vi "Clear.vi"(8 "error in (no error)":errorcluster, 11 "Process In":refnum<class "Process.lvclass">) -> (0 "error out":errorcluster, 3 "Process Out":refnum<class "Process.lvclass">)   [LabVIEW 2020, in "Process.lvclass"]
doc: "Clears any resorces allocated during initialization."
uses:
  Process.lvclass
  Process.lvclass/Process.ctl
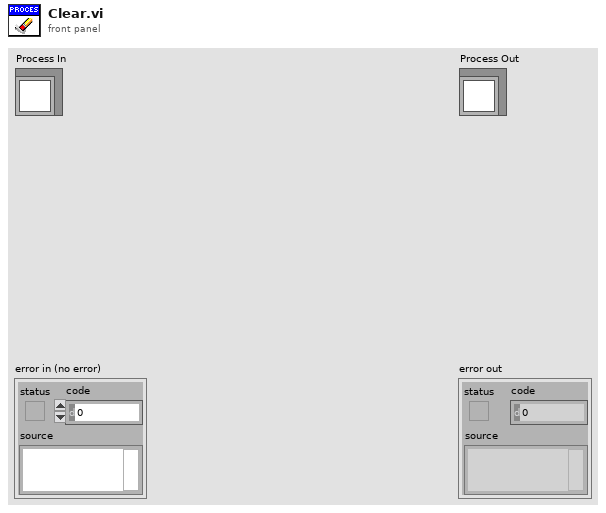
[diagram p1: front panel]
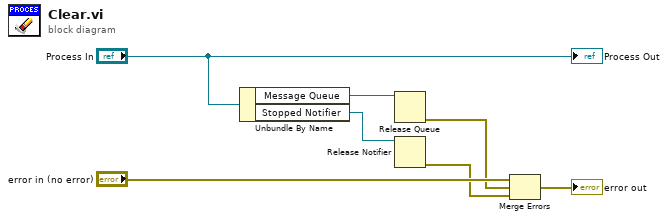
[diagram p0: block diagram]
diagram:
  n1 = Unbundle By Name("Process In") -> ("Message Queue"=w4:refnum<queue>, "Stopped Notifier"=w2:refnum<notifier>)
  n2 = Release Queue(queue=w4) -> (error out=w3:errorcluster)  [unwired: 2 in, 2 out]
  n3 = Release Notifier(notifier=w2) -> (error out=w1:errorcluster)  [unwired: 2 in, 2 out]
  n4 = Merge Errors("error in (no error)", w3, w1) -> (→"error out":errorcluster)
  "Process Out" <- "Process In"
